vi "PH_Beckhoff_StepMot.Action Operation.vi"(0 "VI in":refnum<vi>, 5 "error in":errorcluster) -> (14 "VI out":refnum<vi>, 19 "error out":errorcluster)   [LabVIEW 2014, in "PH_Beckhoff_StepMot.lvlib"]
uses:
  PH_Beckhoff_StepMot.lvlib
  instr.lib/Beckhoff/Beckhoff - Driver np.lvlib
  PH_Beckhoff/PH_Beckhoff.lvlib
  PH_Basics/PH_Stepmotor_BaseClass/PH_Stepmotor_BaseClass.lvlib
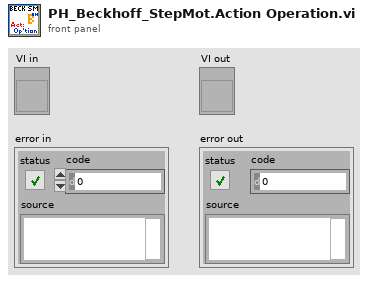
[diagram p1: front panel]
types:
  T1 = typedef "PH_Stepmotor_BaseClass.lvlib/PH_Stepmotor_BaseClass.i attribute.ctl" = cluster{"Device Error":errorcluster, "Axes PSDB Thread":cluster{"Ref":refnum<vi>, "Q-Ref":refnum<queue>, "Data Status":T2}, "Axes":T3[], "Axes PSDB Infos":cluster{"GUI Name":string, "PSDB Instance ID":i32, "PSDB Status Service ID":i32, "Axis":i32, "Class":string}[], "GUI Refs":T8}
  T2 = typedef "PH_PSDBWriter.lvlib/PH_PSDBWriter.Data Status.ctl" = i16
  T3 = typedef "PH_Stepmotor_BaseClass.lvlib/PH_Stepmotor_BaseClass.Axis Attributes.ctl" = cluster{"Settings":T4, "Endswitch?":bool, "DIM Service IDs":T6, "Activity":T7, "Configured?":bool, "Position":cluster{"Current":i32, "Target":i32}, "Position to set":cluster{"New?":bool, "Wanted":i32}, "Stop?":bool, "Reset?":bool, "Move?":bool, "Nothing connected?":bool}
  T4 = typedef "PH_Stepmotor_BaseClass.lvlib/PH_Stepmotor_BaseClass.Axis Settings.ctl" = cluster{"Sign change":bool, "Width":dbl, "Calibration":dbl, "Unit":string, "Motor Type":T5, "Unit Width":string, "Unit CF":string}
  T5 = typedef "PH_Stepmotor_BaseClass.lvlib/PH_Stepmotor_BaseClass.Motor Type.ctl" = enum16{"Unspecific", "OWIS 49.120.2633", "OWIS 49.060.1033", "OWIS 43.040.2558", "Diamond Motion 2200 series", "OWIS 49.120.266B.MV6", "Calorimeter", "Linear Stage 1", "MICOS VT-80", "MICOS VT-80 S", "Standa Rotstage nt0.95A", "PUF RA 320.200", "PUF RA 800.200", "PUF RA 800.400", "PUF RA 400.50", "1324.nn.800.50", "1324.n9c.800.50", "1324.nn.320.200", "1324.nn.400.200", "1324.nn.800.200", "1324.nn.400.50", "1324.8c9c.800.50", "1324.8c9c.400.200"}
  T6 = typedef "PH_Stepmotor_BaseClass.lvlib/PH_Stepmotor_BaseClass.Axis DIM Service IDs.ctl" = cluster{"Settings":i32, "Information":i32}
  T7 = typedef "PH_Stepmotor_BaseClass.lvlib/PH_Stepmotor_BaseClass.Axis Activity.ctl" = enum16{"No Information", "stopped", "running", "Failure", "Alarm", "stopped at backward ES", "stopped at foreward ES"}
  T8 = typedef "PH_Stepmotor_BaseClass.lvlib/PH_Stepmotor_BaseClass.GUI Refs.ctl" = cluster{"Axes Configuration":refnum<vi>, "Device Error":refnum<vi>, "Axes PSDB Infos":refnum<vi>}
  T9 = typedef "PH_Beckhoff.lvlib/PH_Beckhoff.i attribute.ctl" = cluster{"GUI Refs":T10, "operation?":bool, "Default Prdc Interval":i32, "Connection":T11, "AMS Net ID":T12, "Klemmencluster: # of":T13, "Values":T14, "IP":string, "Description":string, "configured?":bool, "Change Manager":cluster{"Detemination wanted?":bool, "Values changed at":cluster{"Sonderklemmen Inputs":i32[], "Analog Inputs":i32[], "Analog Outputs":i32[], "Digital Inputs":i32[], "Digital Outputs":i32[]}}, "Difference to handle an analog input as change":u32}
  T10 = typedef "PH_Beckhoff.lvlib/PH_Beckhoff.GUI Refs.ctl" = cluster{"ADS Error":refnum<vi>, "Values":refnum<vi>, "configured?":refnum<vi>, "Connection":refnum<vi>, "IP":refnum<vi>, "Prdc Int [ms]":refnum<vi>}
  T11 = typedef "PH_Beckhoff.lvlib/PH_Beckhoff.Connectivity.ctl" = cluster{"DLL?":bool, "Port?":bool, "Client?":bool, "Ping?":bool, "unsuccessful Pings":u32}
  T12 = typedef "Beckhoff - Driver np.lvlib/Beckhoff Access.ctl" = cluster{"DLL path":path, "AMS Net ID":cluster{"1st # of IP":u8, "2nd # of IP":u8, "3rd # of IP":u8, "4th # of IP":u8, "In Port":u8, "Out Port":u8}}
  T13 = typedef "Beckhoff - Driver np.lvlib/Klemmendeclarer.ctl" = cluster{"Offset due to Sonderklemms":u32, "analog Inputs":u32, "analog Outputs":u32, "digital Input Bits":u32, "digital Output Bits":u32}
  T14 = typedef "PH_Beckhoff.lvlib/PH_Beckhoff.Values.ctl" = cluster{"Sonderklemmen Inputs":T15, "Analog Inputs":T16, "Analog Outputs":T18, "Digital Inputs":T19, "Digital Outputs":T20}
  T15 = typedef "PH_Beckhoff.lvlib/PH_Beckhoff.Sonderklemmen Inputs.ctl" = cluster{"Total Length":u32, "Name":string, "Value":u64, "Quality":bool, "Service ID":i32, "Offset":u32, "Length":u32}[]
  T16 = typedef "PH_Beckhoff.lvlib/PH_Beckhoff.Analog Inputs.ctl" = cluster{"Name":string, "Value":u32, "Quality":bool, "Service ID":i32, "Sca Type":T17}[]
  T17 = typedef "PH_Beckhoff.lvlib/PH_Beckhoff.Scaling Type.ctl" = enum16{"none", "0 ... 15 Bit -> 0 ... 5", "0 ... 15 Bit -> 0 ... 10", "0 ... 15 Bit -> 0 ... 25", "0 ... 15 Bit -> 4 ... 20", "0 ... 15 Bit -> 0 ... 1", "0 ... 15 Bit -> 0 ... 20000", "0 ... 15 Bit -> 0 ... 24000"}
  T18 = typedef "PH_Beckhoff.lvlib/PH_Beckhoff.Analog Outputs.ctl" = cluster{"Name":string, "Value":u32, "Quality":bool, "Wanted Value":u32, "Service ID":i32, "Sca Type":T17}[]
  T19 = typedef "PH_Beckhoff.lvlib/PH_Beckhoff.Digital Inputs.ctl" = cluster{"Name":string, "Value":bool, "Quality":bool, "Service ID":i32, "inverted?":bool}[]
  T20 = typedef "PH_Beckhoff.lvlib/PH_Beckhoff.Digital Outputs.ctl" = cluster{"Name":string, "Value":bool, "Quality":bool, "Wanted Value":bool, "Service ID":i32, "inverted?":bool}[]
  T21 = typedef "PH_Beckhoff_StepMot.lvlib/PH_Beckhoff_StepMot.i attribute.ctl" = cluster{"Axes Settings":T22[], "GUI Refs":cluster{"Axes Settings":refnum<vi>, "Stati":refnum<vi>}, "Get Beckhoff Settings":bool}
  T22 = typedef "PH_Beckhoff_StepMot.lvlib/PH_Beckhoff_StepMot.Axis Cluster.ctl" = cluster{"Step Motor Configuration":T23, "To set?":bool, "Endswitch inverted?":bool}
  T23 = typedef "Beckhoff - Driver np.lvlib/Beckhoff.Step Motor - Motor Configuration.ctl" = cluster{"Feature Register":T24, "I max A [mA]":dbl, "I max B [mA]":dbl, "v min":u32, "v max":u32, "a max":u32, "I hold [%]":u32, "Steps/qp":u32, "Feature Register 2":T25}
  T24 = typedef "Beckhoff - Driver np.lvlib/Beckhoff.Step Motor - Feature Register 1.ctl" = cluster{"en Auto Start":bool, "en Auto Stop":bool, "dis Wd Timer":bool, "OP Mode 1":bool, "OP Mode 2":bool, "Ramp Type":bool, "inv Pos Feedback":bool, "en User Cur Table":bool, "en Latch Evt Clr Pos":bool, "en Multi Latch Vals":bool, "en Sign Disp*":bool, "Feedback Type*":bool, "en neg Gate Lock*":bool, "en pos Gate Lock*":bool, "dis Enc Fltr*":bool, "en Counter Mode*":bool}
  T25 = typedef "Beckhoff - Driver np.lvlib/Beckhoff.Step Motor - Feature Register 2.ctl" = cluster{"rev Homing Dir":bool, "en Decac Ramp":bool, "Latch Reg Pos":bool, "Show Idle":bool, "dis Ref Input 1":bool, "dis Ref Input 2":bool, "en ext Auto Start":bool, "N/A":bool, "N/A":bool, "N/A":bool, "N/A":bool, "N/A":bool, "en Clr Proc Data":bool, "en Man Ecl Tolerce*":bool, "rev Dig Input 1":bool, "rev Dig Input 2":bool}
  T26 = typedef "Beckhoff - Driver np.lvlib/Beckhoff.Step Motor - Status.ctl" = cluster{"Byte":T27, "Word":T28}
  T27 = typedef "Beckhoff - Driver np.lvlib/Beckhoff.Step Motor - Status Byte.ctl" = cluster{"Ready":bool, "Load Angle 1":bool, "Load Angle 2":bool, "Load Angle 3":bool, "Idle":bool, "Warning":bool, "Error":bool, "RegAccess":bool}
  T28 = typedef "Beckhoff - Driver np.lvlib/Beckhoff.Step Motor - Status Word.ctl" = cluster{"Input 1":bool, "Input 2":bool, "Set Pos Ready":bool, "Target reached":bool, "Latch valid":bool, "Latch Data InByte 2,3":bool, "Latch Data toggled":bool, "Eencoder disabled":bool, "Over temperature":bool, "Under voltage":bool, "Open load Br A":bool, "Open load Br B":bool, "Over current Br A":bool, "Over current Br B":bool, "No control Power":bool, "Config Error":bool}
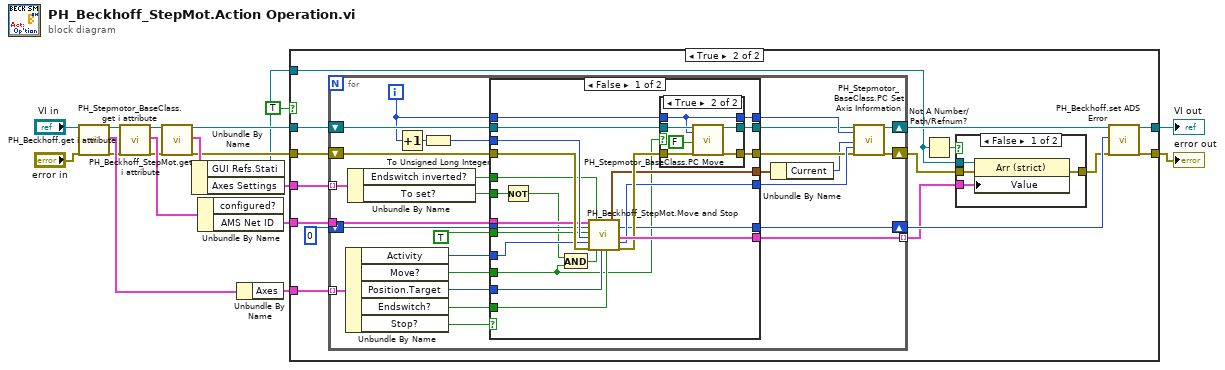
[diagram p0: block diagram]
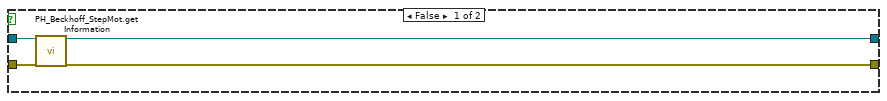
[diagram p2: hidden frame]
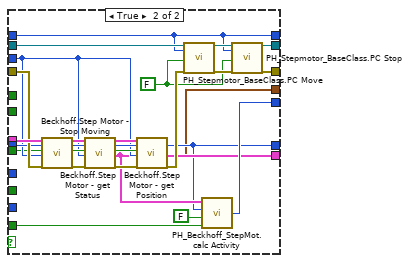
[diagram p5: hidden frame]
diagram:
  n1 = call "PH_Stepmotor_BaseClass.get i attribute.vi"("i ref in"="VI in", "error in (no error)"="error in") -> ("i ref out"=w6:refnum<vi>, "i attribute"=w12:T1, "error out"=w4:errorcluster)  [unwired: 15 in]
  n2 = call "PH_Beckhoff.get i attribute.vi"("i ref in"=w6, "error in (no error)"=w4) -> ("i ref out"=w5:refnum<vi>, "i attribute"=w16:T9, "error out"=w3:errorcluster)  [unwired: 15 in]
  n3 = call "PH_Beckhoff_StepMot.get i attribute.vi"("i ref in"=w5, "error in (no error)"=w3) -> ("i ref out"=w8:refnum<vi>, "i attribute"=w14:T21, "error out"=w7:errorcluster)  [unwired: 15 in]
  n4 = Unbundle By Name(w14) -> ("GUI Refs.Stati"=w2:refnum<vi>, "Axes Settings"=w13:T22[])
  n5 = Unbundle By Name(w16) -> ("AMS Net ID"=w15:T12)  [unwired: 1 out]
  n6 = Unbundle By Name(w12) -> ("Axes"=w11:T3[])
  n7 = case shown="True" TRUE {
    tunnel: [w19 w34] -> w18
    tunnel: [w21 w33] -> w17
    tunnel: w8 -> [w20 w37]
    tunnel: w15 -> [_ w30]
    tunnel: w7 -> [w22 w28]
    tunnel: w13 -> [_ w31]
    tunnel: w11 -> [_ w36]
    tunnel: w2 -> [_ w24]
    frame False {
      n8 = call "PH_Beckhoff_StepMot.get Information.vi"("VI in"=w20, "error in"=w22) -> ("VI out"=w19:refnum<vi>, "error out"=w21:errorcluster)  [unwired: 16 in]
    }
    frame True {
      n9 = for {
        tunnel: w30 -> [w60]
        shift-right: [w54] -> w35
        shift-left: w37 -> [w64]
        shift-right: [w53] -> w23
        shift-left: w28 -> [w58]
        tunnel: w31 -> [w65] mode=indexing
        shift-right: [w52] -> w32
        shift-left: 0 ("ADS Error out") -> [w59]
        tunnel: w36 -> [w68] mode=indexing
        tunnel: [w56] -> w25 mode=indexing
        i -> [w61]
        n10 = Unbundle By Name(w68) -> ("Activity"=w47:T7, "Move?"=w48:bool, "Position.Target"=w66:i32, "Endswitch?"=w67:bool, "Stop?"=w63:bool)
        n11 = Unbundle By Name(w65) -> ("Endswitch inverted?"=w44:bool, "To set?"=w43:bool)
        n12 = Increment(x=w61) -> (x+1=w69:i32)
        n13 = To Unsigned Long Integer(number=w69) -> (unsigned 32bit integer=w62:u32)
        n14 = case shown="False" w63 {
          tunnel: w60 -> [w80 w128]
          tunnel: w58 -> [w85 w127]
          tunnel: [w91 w115] -> w49
          tunnel: w62 -> [w87 w109]
          tunnel: [w81 w106] -> w52
          tunnel: w59 -> [w79 w126]
          tunnel: w67 -> [w77 w105]
          tunnel: w66 -> [w78 _]
          tunnel: w48 -> [w71 _]
          tunnel: TRUE ("Read?") -> [w84 w102]
          tunnel: w44 -> [w74 _]
          tunnel: w61 -> [w90 w112]
          tunnel: w64 -> [w88 w125]
          tunnel: [w92 w113] -> w50
          tunnel: [w89 w112] -> w55
          tunnel: [w86 w107] -> w56
          tunnel: [w82 w108] -> w51
          tunnel: w47 -> [w76 _]
          tunnel: [w75 w103] -> w46
          tunnel: w43 -> [w73 _]
          frame False {
            n15 = Not(x=w73) -> (.not. x?=w72:bool)
            n16 = And(x=w72, y=w71) -> (x .and. y?=w70:bool)
            n17 = call "PH_Beckhoff_StepMot.Move and Stop.vi"("AMS Net ID in"=w80, "ADS Error in"=w79, "Read and Write?"=w84, "# of Klemme [1, ...]"=w87, "Axis Activity in"=w76, "error in (no error)"=w85, "Endswitch inverted?"=w74, "Move?"=w70, "Target"=w78, "Endswitch?"=w77) -> ("Position"=w75:cluster{"Target":i32, "Current":i32}, "ADS Error out"=w81:i32, "Status"=w86:T26, "Axis Activity out"=w82:T7, "error out"=w83:errorcluster)  [unwired: 3 in, 2 out]
            n18 = case shown="True" w71 {
              tunnel: w88 -> [w94 w101]
              tunnel: [w94 w100] -> w92
              tunnel: w83 -> [w93 w99]
              tunnel: [w93 w98] -> w91
              tunnel: w90 -> [w95 w96]
              tunnel: [w95 w96] -> w89
              frame False {
              }
              frame True {
                n19 = call "PH_Stepmotor_BaseClass.PC Move.vi"("i ref in"=w101, "axis"=w96, "Move"=FALSE, "error in (no error)"=w99) -> ("i ref out"=w100:refnum<vi>, "error out"=w98:errorcluster)  [unwired: 14 in]
              }
            }
          }
          frame True {
            w111 = FALSE ("Move")
            n20 = call "Beckhoff.Step Motor - Stop Moving.vi"("AMS Net ID in"=w128, "ADS Error in (0)"=w126, "Write?"=w102, "Klemme"=w109, "error in (no error)"=w127) -> ("AMS Net ID out"=w120:T12, "ADS Error out"=w119:i32, "Write successful?"=w110:bool, "error out"=w118:errorcluster)  [unwired: 11 in]
            n21 = call "Beckhoff.Step Motor - get Status.vi"("AMS Net ID in"=w120, "ADS Error in (0)"=w119, "Read?"=w110, "# of Klemme [1, ...]"=w109, "error in (no error)"=w118) -> ("AMS Net ID out"=w123:T12, "ADS Error out"=w122:i32, "Read successful?"=w121:bool, "Status"=w107:T26, "error out"=w116:errorcluster)  [unwired: 10 in]
            n22 = call "Beckhoff.Step Motor - get Position.vi"("AMS Net ID in"=w123, "ADS Error in (0)"=w122, "Read?"=w121, "# of Klemme [1, ...]"=w109, "error in (no error)"=w116) -> ("ADS Error out"=w106:i32, "Position"=w103:cluster{"Target":i32, "Current":i32}, "error out"=w117:errorcluster)  [unwired: 10 in, 2 out]
            n23 = call "PH_Stepmotor_BaseClass.PC Move.vi"("i ref in"=w125, "axis"=w112, "Move"=w111, "error in (no error)"=w117) -> ("i ref out"=w114:refnum<vi>, "error out"=w124:errorcluster)  [unwired: 14 in]
            n24 = call "PH_Beckhoff_StepMot.calc Activity.vi"("Endswitch?"=w105, "Moving"=FALSE, "ADS Error in"=w106, "Status"=w107) -> ("Axis Activity"=w108:T7)
            n25 = call "PH_Stepmotor_BaseClass.PC Stop.vi"("i ref in"=w114, "axis"=w112, "Stop"=w111, "error in (no error)"=w124) -> ("i ref out"=w113:refnum<vi>, "error out"=w115:errorcluster)  [unwired: 14 in]
          }
        }
        n26 = Unbundle By Name(w46) -> ("Current"=w45:i32)
        n27 = call "PH_Stepmotor_BaseClass.PC Set Axis Information.vi"("i ref in"=w50, "axis"=w55, "Current Position (Steps)"=w45, "Axis Activity"=w51, "error in (no error)"=w49) -> ("i ref out"=w54:refnum<vi>, "error out"=w53:errorcluster)  [unwired: 13 in]
      }
      n28 = Not A Number/Path/Refnum?(number/path/refnum=w24) -> (NaN/Path/Refnum?=w27:bool)
      n29 = case shown="False" w27 {
        tunnel: w23 -> [w41 w42]
        tunnel: [w40 w42] -> w26
        tunnel: w24 -> [w39 _]
        tunnel: w25 -> [w38 _]
        frame False {
          n30 = property class="Arr (strict)"(reference=w39, error in=w41, "Value"=w38) -> (error out=w40:errorcluster)  [unwired: 1 out]
        }
        frame True {
        }
      }
      n31 = call "PH_Beckhoff.set ADS Error.vi"("i ref in"=w35, "ADS Error"=w32, "error in"=w26) -> ("i ref out"=w34:refnum<vi>, "error out"=w33:errorcluster)  [unwired: 15 in]
    }
  }
  "VI out" <- w18
  "error out" <- w17
